vi "BRig_dataTrial_iTrial_PostR.vi"() -> (2 "output_iTrial_PostR":i32)   [LabVIEW 2014]
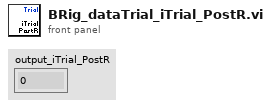
[diagram p1: front panel]
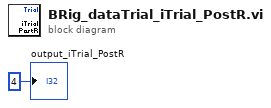
[diagram p0: block diagram]
diagram:
  "output_iTrial_PostR" <- 4 ("output_iBlock")
